vi "verify acquisition parameters in range.vi"(8 "error in (no error)":errorcluster, 11 "Simulated_CCD_Camera in":refnum<class "Simulated Camera.lvclass">) -> (0 "error out":errorcluster, 3 "Simulated_CCD_Camera out":refnum<class "Simulated Camera.lvclass">)   [LabVIEW 2018, in "Simulated Camera.lvclass"]
doc: "Verify if the parameters of the camera are in range\n\nThe operating parameters of the CCDs must be within a predefined range. This function verifies if the values provided for these parameters meet this specification. If not, ACS will not allow to start an exposure."
uses:
  Simulated Camera.lvclass
panel:
  out "New SET parameters 2":T1
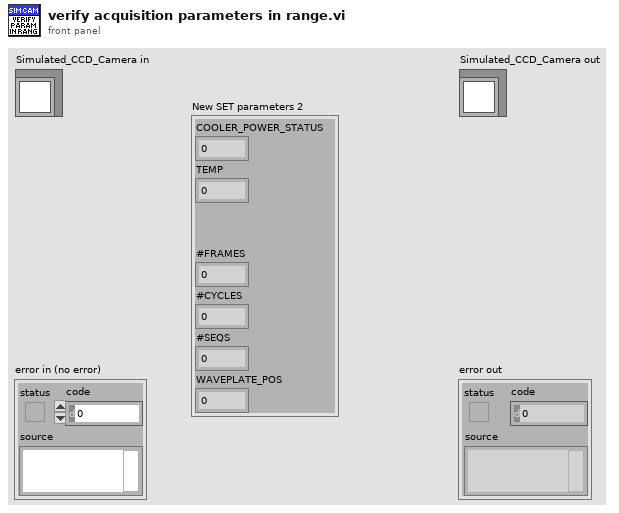
[diagram p1: front panel]
types:
  T1 = cluster{"COOLER_POWER_STATUS":u16, "TEMP":i32, "#FRAMES":u32, "#CYCLES":u32, "#SEQS":u32, "WAVEPLATE_POS":u16}
  T2 = cluster{"COOLER_POWER_STATUS":u16, "TEMP":i32, "EXPTIME":dbl, "#FRAMES":u32, "#CYCLES":u32, "#SEQS":u32, "WAVEPLATE_POS":u16}
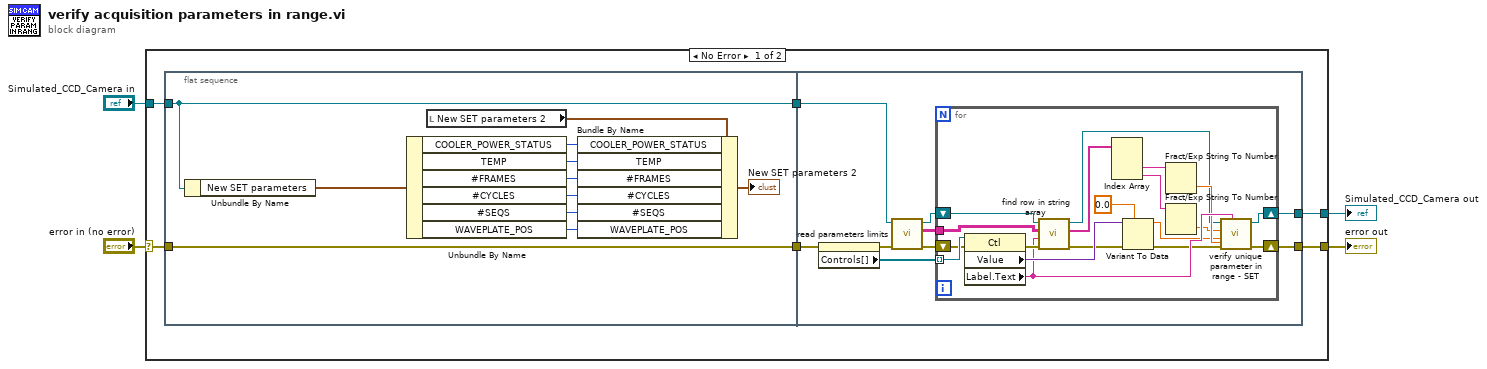
[diagram p0: block diagram]
diagram:
  n1 = case shown="No Error" "error in (no error)" {
    selector: "error in (no error)" -> [w8 w51]
    tunnel: [w10 w51] -> w3
    tunnel: [w9 w50] -> w2
    tunnel: "Simulated_CCD_Camera in" -> [w7 w50]
    frame No Error {
      n2 = flat-sequence {
        tunnel: w7 -> [w20]
        tunnel: w8 -> [w21]
        tunnel: [w21] -> w6
        tunnel: [w20] -> w5
        tunnel: [w30] -> w10
        tunnel: [w29] -> w9
        tunnel: w6 -> [w23]
        tunnel: w5 -> [w25]
        frame #0 {
          n3 = Unbundle By Name(w20) -> ("New SET parameters"=w17:T2)
          n4 = Unbundle By Name(w17) -> ("COOLER_POWER_STATUS"=w16:u16, "TEMP"=w15:i32, "#FRAMES"=w14:u32, "#CYCLES"=w13:u32, "#SEQS"=w12:u32, "WAVEPLATE_POS"=w11:u16)
          n5 = local read "New SET parameters 2"() -> (w19:T1)
          n6 = Bundle By Name(cluster=w19, "COOLER_POWER_STATUS"=w16, "TEMP"=w15, "#FRAMES"=w14, "#CYCLES"=w13, "#SEQS"=w12, "WAVEPLATE_POS"=w11) -> (→"New SET parameters 2":T1)
        }
        frame #1 {
          n7 = property on="New SET parameters 2" class="Clust (strict)"(error in=w23) -> (error out=w22:errorcluster, "Controls[]"=w24:refnum<vi>[])  [unwired: 1 in, 1 out]
          n8 = call "read parameters limits.vi"("error in (no error)"=w22, "Simulated_CCD_Camera in"=w25) -> ("error out"=w28:errorcluster, "limit values spreadsheet"=w27:string[][], "Simulated_CCD_Camera out"=w26:refnum<class "Simulated Camera.lvclass">)  [unwired: 7 in]
          n9 = for {
            shift-right: [w34] -> w30
            shift-left: w28 -> [w39]
            tunnel: w24 -> [w49] mode=indexing
            tunnel: w27 -> [w46]
            shift-right: [w33] -> w29
            shift-left: w26 -> [w44]
            n10 = property class="Ctl"(reference=w49, error in=w39) -> (error out=w41:errorcluster, "Value"=w48:variant, "Label.Text"=w38:string)  [unwired: 1 out]
            n11 = call "find row in string array.vi"("error in (no error)"=w41, "parameter name"=w38, "limit values"=w46, "Simulated_CCD_Camera in"=w44) -> ("error out"=w40:errorcluster, "row"=w45:string[], "Simulated_CCD_Camera out"=w32:refnum<class "Simulated Camera.lvclass">)  [unwired: 5 in]
            n12 = Index Array(array=w45) -> (element #2=w43:string, element #3=w42:string)  [unwired: 3 in, 1 out]
            n13 = Variant To Data(error in=w40, type=0.0, Variant=w48) -> (data=w36:dbl, error out=w31:errorcluster)
            n14 = Fract/Exp String To Number(string=w43) -> (number=w37:dbl)  [unwired: 3 in, 1 out]
            n15 = Fract/Exp String To Number(string=w42) -> (number=w35:dbl)  [unwired: 3 in, 1 out]
            n16 = call "verify unique parameter in range - SET.vi"(6:w37, 7:w38, "error in (no error)"=w31, "value"=w36, "parameter name"=w35, "Simulated_CCD_Camera in"=w32) -> ("error out"=w34:errorcluster, "Simulated_CCD_Camera out"=w33:refnum<class "Simulated Camera.lvclass">)  [unwired: 4 in]
          }
        }
      }
    }
    frame Error {
    }
  }
  "error out" <- w3
  "Simulated_CCD_Camera out" <- w2
